vi "_Get Mass Dependent Parameters.vi"(4 "error in (no error)":errorcluster, 7 "node in":refnum<k20>) -> (0 "error out":errorcluster, 2 "Parameters":T1[](array[typedef]), 3 "node out":refnum<k20>)   [LabVIEW 2015]
uses:
  Type/_Mass Range Parameters.ctl
  <vilib>/xml/Close Reference(Node).vi
  <vilib>/xml/NI_XML.lvlib
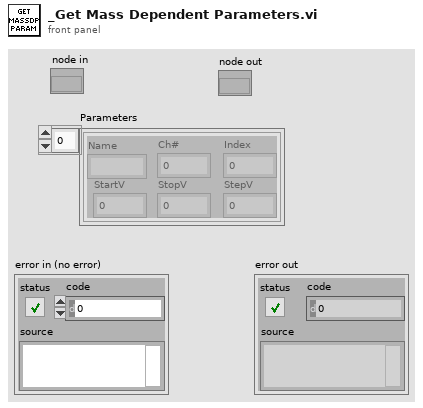
[diagram p1: front panel]
types:
  T1 = typedef "_Mass Range Parameters.ctl" = cluster{"Name":string, "Ch#":u8, "StartV":dbl, "StopV":dbl, "StepV":dbl, "Index":u8}
  T2 = typedef "_RT Configuration 2.ctl" = cluster{"Name":string, "Ch#":u8, "Min":dbl, "Max":dbl, "Def+":dbl, "Def-":dbl, "Offset":dbl, "Slope":dbl, "Type":u8, "Description":string, "SettleT":dbl}
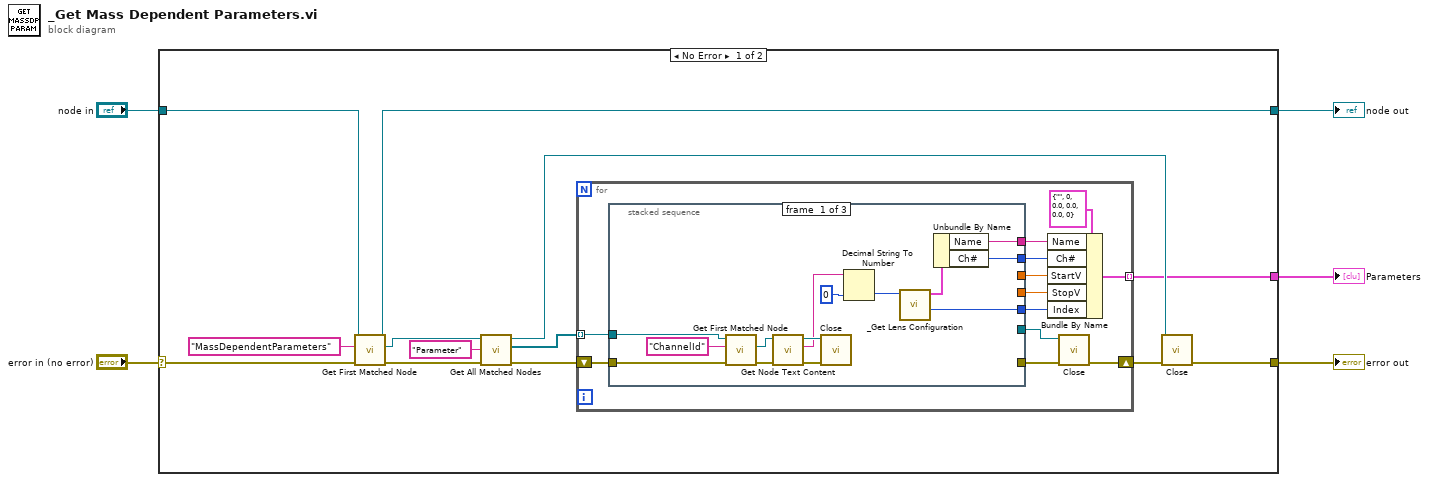
[diagram p0: block diagram]
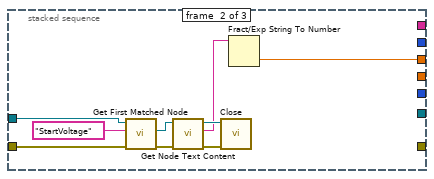
[diagram p2: hidden frame]
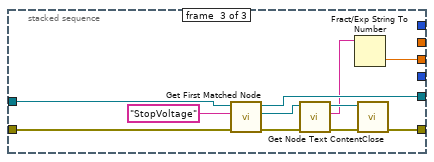
[diagram p3: hidden frame]
diagram:
  n1 = case shown="No Error" "error in (no error)" {
    selector: "error in (no error)" -> [w15 w65]
    tunnel: "node in" -> [w16 w66]
    tunnel: [w14 w66] -> w3
    tunnel: [w9 w65] -> w2
    tunnel: [w6 _] -> w1
    frame No Error {
      n2 = call <vilib>:"Get First Matched Node.vi"("error in (no error)"=w15, "XPath expression"="MassDependentParameters", "node in"=w16) -> ("error out"=w12:errorcluster, "node result"=w13:refnum<k20>, "node out"=w14:refnum<k20>)  [unwired: 6 in]
      n3 = call <vilib>:"Get All Matched Nodes.vi"("error in (no error)"=w12, "XPath expression"="Parameter", "node in"=w13) -> ("error out"=w7:errorcluster, "node result array"=w8:refnum<k20>[], "node out"=w10:refnum<k20>)  [unwired: 6 in]
      n4 = for {
        shift-right: [w28] -> w11
        shift-left: w7 -> [w29]
        tunnel: w8 -> [w30] mode=indexing
        tunnel: [w25] -> w6 mode=indexing
        n5 = stacked-sequence {
          tunnel: w30 -> [w44 w53 w64]
          tunnel: w29 -> [w43 w52 w63]
          tunnel: [_ _ w57] -> w27
          tunnel: [_ _ w56] -> w26
          tunnel: [w33 _ _] -> w24
          tunnel: [w32 _ _] -> w23
          tunnel: [_ w45 _] -> w22
          tunnel: [_ _ w54] -> w21
          tunnel: [w31 _ _] -> w20
          frame #0 {
            n6 = call <vilib>:"Get First Matched Node.vi"("error in (no error)"=w43, "XPath expression"="ChannelId", "node in"=w44) -> ("error out"=w38:errorcluster, "node result"=w41:refnum<k20>)  [unwired: 6 in, 1 out]
            n7 = call <vilib>:"Get Node Text Content.vi"("error in (no error)"=w38, "node in"=w41) -> ("error out"=w39:errorcluster, "node text"=w37:string, "node out"=w40:refnum<k20>)  [unwired: 7 in]
            n8 = call-poly <vilib>:"Close.vi"("error in (no error)"=w39, "node"=w40) -> ()  [unwired: 7 in, 1 out]
            n9 = Decimal String To Number(string=w37, default (0L)=u8 0 ("default (0 I32)")) -> (number=w35:u8)  [unwired: 1 in, 1 out]
            n10 = call "_Get Lens Configuration.vi"("Channel #"=w35) -> ("Config Row#"=w31:i32, "Lens Configuration"=w34:T2)  [unwired: 1 in, 4 out]
            n11 = Unbundle By Name(w34) -> ("Name"=w33:string, "Ch#"=w32:u8)
          }
          frame #1 {
            n12 = call <vilib>:"Get First Matched Node.vi"("error in (no error)"=w52, "XPath expression"="StartVoltage", "node in"=w53) -> ("error out"=w49:errorcluster, "node result"=w50:refnum<k20>)  [unwired: 6 in, 1 out]
            n13 = call <vilib>:"Get Node Text Content.vi"("error in (no error)"=w49, "node in"=w50) -> ("error out"=w48:errorcluster, "node text"=w46:string, "node out"=w47:refnum<k20>)  [unwired: 7 in]
            n14 = call-poly <vilib>:"Close.vi"("error in (no error)"=w48, "node"=w47) -> ()  [unwired: 7 in, 1 out]
            n15 = Fract/Exp String To Number(string=w46) -> (number=w45:dbl)  [unwired: 3 in, 1 out]
          }
          frame #2 {
            n16 = call <vilib>:"Get First Matched Node.vi"("error in (no error)"=w63, "XPath expression"="StopVoltage", "node in"=w64) -> ("error out"=w60:errorcluster, "node result"=w61:refnum<k20>, "node out"=w57:refnum<k20>)  [unwired: 6 in]
            n17 = call <vilib>:"Get Node Text Content.vi"("error in (no error)"=w60, "node in"=w61) -> ("error out"=w59:errorcluster, "node text"=w55:string, "node out"=w58:refnum<k20>)  [unwired: 7 in]
            n18 = Fract/Exp String To Number(string=w55) -> (number=w54:dbl)  [unwired: 3 in, 1 out]
            n19 = call-poly <vilib>:"Close.vi"("error in (no error)"=w59, "node"=w58) -> ("error out"=w56:errorcluster)  [unwired: 7 in]
          }
        }
        n20 = Bundle By Name(cluster=T1 {"Name"="", "Ch#"=0, "StartV"=0.0, "StopV"=0.0, "StepV"=0.0, "Index"=0} ("MR Parameters"), "Name"=w24, "Ch#"=w23, "StartV"=w22, "StopV"=w21, "Index"=w20) -> (w25:T1)
        n21 = call-poly <vilib>:"Close.vi"("error in (no error)"=w26, "node"=w27) -> ("error out"=w28:errorcluster)  [unwired: 7 in]
      }
      n22 = call-poly <vilib>:"Close.vi"("error in (no error)"=w11, "node"=w10) -> ("error out"=w9:errorcluster)  [unwired: 7 in]
    }
    frame Error {
    }
  }
  "error out" <- w2
  "node out" <- w3
  "Parameters" <- w1
